vi "getUnits.vi"(8 "error in (no error)":errorcluster, 11 "RfOutputChannel.lvclass in":refnum<class "RfOutputChannel.lvclass">) -> (0 "error out":errorcluster, 2 "units":string, 3 "RfOutputChannel.lvclass out":refnum<class "RfOutputChannel.lvclass">)   [LabVIEW 2011, in "Tools.lvlib" / "DatabaseHelpers.lvlib" / "RfOutputChannel.lvclass"]
uses:
  RfOutputChannel.lvclass
  RfOutputChannel.lvclass/RfOutputChannel.ctl
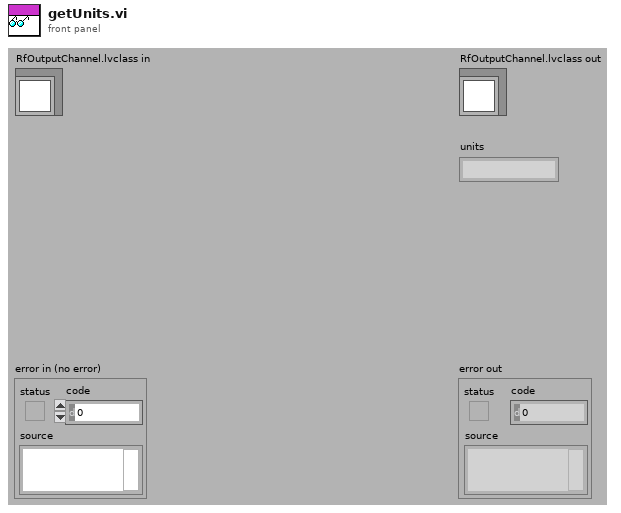
[diagram p1: front panel]
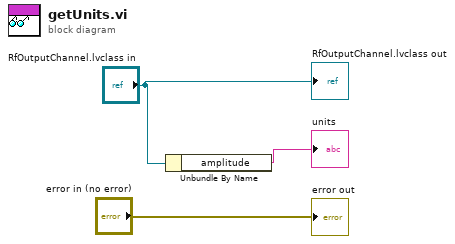
[diagram p0: block diagram]
diagram:
  n1 = Unbundle By Name("RfOutputChannel.lvclass in") -> ("amplitude"=→"units":string)
  "error out" <- "error in (no error)"
  "RfOutputChannel.lvclass out" <- "RfOutputChannel.lvclass in"
